vi "On Click Enumerate Cameras.vi"(8 "error in (no error)":errorcluster, 10 "Value":bool, 11 "App in":refnum<class "App.lvclass">) -> (0 "error out":errorcluster, 3 "App out":refnum<class "App.lvclass">)   [LabVIEW 2020, in "AR Example.lvlib" / "App.lvclass"]
uses:
  App.lvclass
  App.lvclass/App.ctl
  UI/UI.lvclass
  b0e96125-61a1-4303-b342-3e2cae2d3e9f.vi
  917a6586-ad63-4fd0-8dd0-0daf31f14cd0.vi
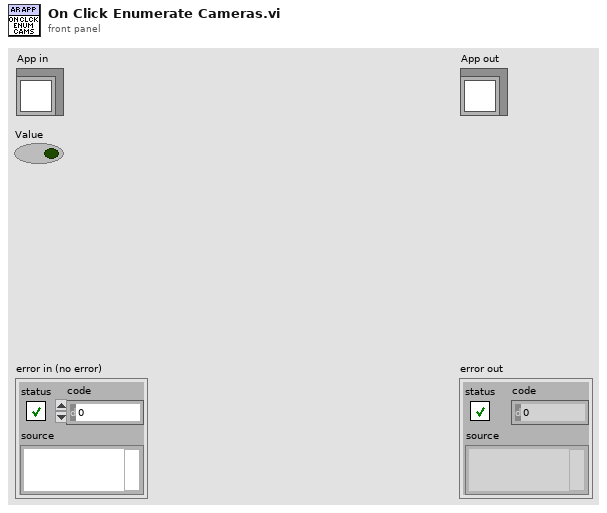
[diagram p1: front panel]
types:
  T1 = enum16{"Set UI Pre Enum", "Enumerate", "Update Lists", "Set UI Post Enum"}
  T2 = enum16{"Set UI Pre Enum", "Enumerate", "Update Lists", "Set UI Post Enum"}[]
  T3 = typedef "g_ar_toolkit.capture.lvlib/Stream.lvclass/Device Enumeration.ctl" = cluster{"Name":string, "Streams":set{T4}}
  T4 = typedef "g_ar_toolkit.capture.lvlib/Stream.lvclass/Stream Parameters.ctl" = cluster{"Width":u16, "Height":u16, "FPS":u8}
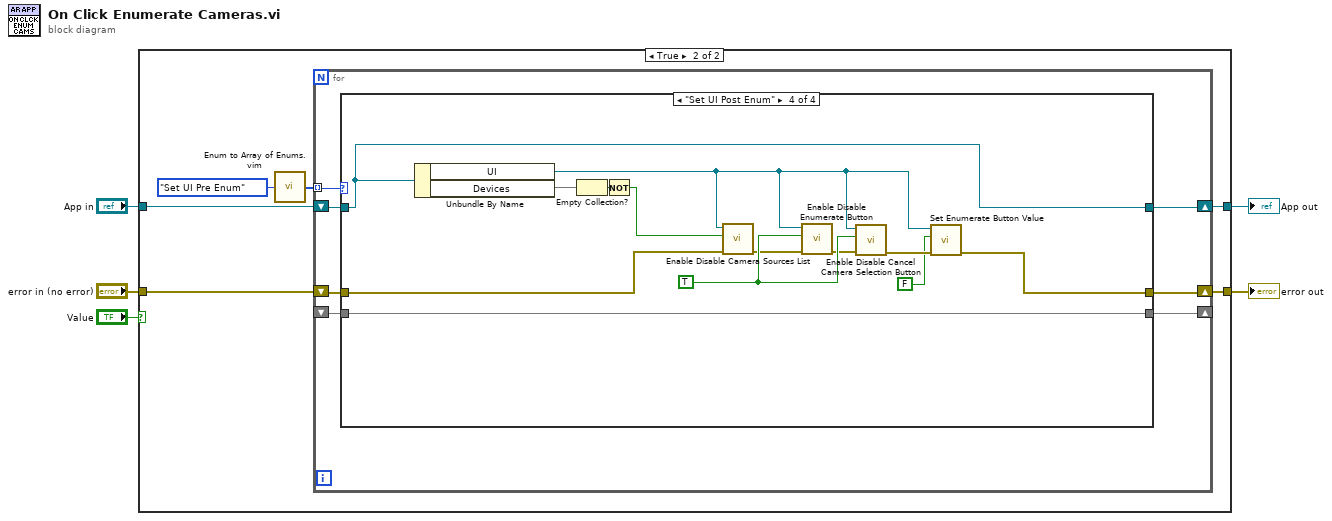
[diagram p0: block diagram]
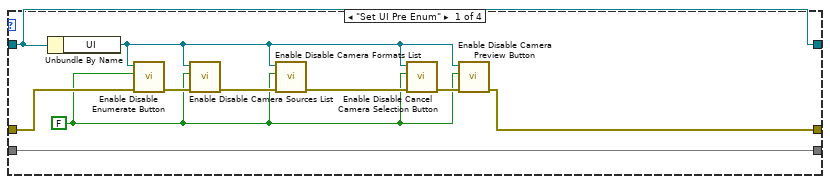
[diagram p3: hidden frame]
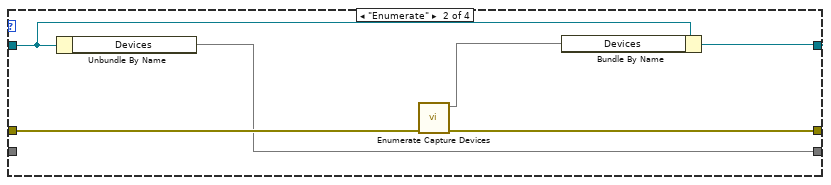
[diagram p4: hidden frame]
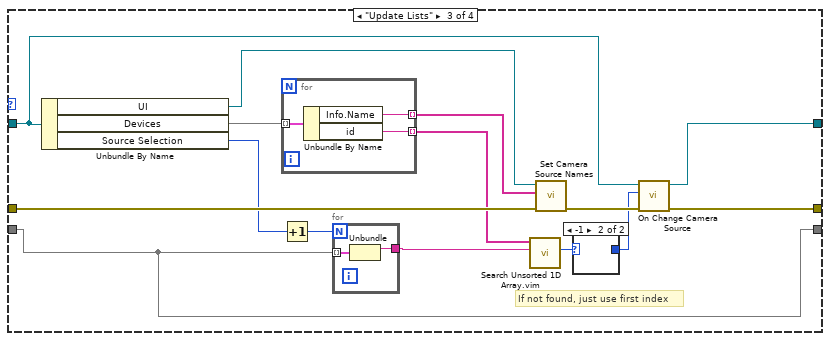
[diagram p5: hidden frame]
diagram:
  n1 = case shown="True" "Value" {
    tunnel: "App in" -> [w6 w13]
    tunnel: "error in (no error)" -> [w7 w12]
    tunnel: [w7 w11] -> w3
    tunnel: [w6 w10] -> w2
    frame False {
    }
    frame True {
      n2 = call "Enum to Array of Enums.vim"("enum"=T1."Set UI Pre Enum") -> ("array of enums"=w8:T2)
      n3 = for {
        shift-right: [w19] -> w11
        shift-left: w12 -> [w20]
        shift-right: [w16] -> w10
        shift-left: w13 -> [w18]
        tunnel: w8 -> [w17] mode=indexing
        shift-right: [w15] -> _
        shift-left: _ -> [w14]
        n4 = case shown="\"Set UI Post Enum\"" w17 {
          tunnel: w20 -> [w30 w36 w49 w60]
          tunnel: [w21 w33 w43 w64] -> w19
          tunnel: w18 -> [w26 w35 w45 w69]
          tunnel: [w26 w34 w44 w69] -> w16
          tunnel: [w25 w32 w51 w68] -> w15
          tunnel: w14 -> [w25 _ w51 w68]
          frame "Set UI Pre Enum" {
            w22 = FALSE ("Enable?")
            n5 = Unbundle By Name(w26) -> ("UI"=w23:refnum<class "UI.lvclass">)
            n6 = call-dynamic "Enable Disable Enumerate Button.vi"("error in (no error)"=w30, "Enable?"=w22, "UI in"=w23) -> ("error out"=w29:errorcluster)  [unwired: 8 in]
            n7 = call-dynamic "Enable Disable Camera Sources List.vi"("error in (no error)"=w29, "Enable?"=w22, "UI in"=w23) -> ("error out"=w28:errorcluster)  [unwired: 8 in]
            n8 = call-dynamic "Enable Disable Camera Formats List.vi"("error in (no error)"=w28, "Enable?"=w22, "UI in"=w23) -> ("error out"=w27:errorcluster)  [unwired: 8 in]
            n9 = call-dynamic "Enable Disable Cancel Camera Selection Button.vi"("error in (no error)"=w27, "Enable?"=w22, "UI in"=w23) -> ("error out"=w24:errorcluster)  [unwired: 8 in]
            n10 = call-dynamic "Enable Disable Camera Preview Button.vi"("error in (no error)"=w24, "Enable?"=w22, "UI in"=w23) -> ("error out"=w21:errorcluster)  [unwired: 8 in]
          }
          frame "Enumerate" {
            n11 = Unbundle By Name(w35) -> ("Devices"=w32:map{string, T3})
            n12 = call "Enumerate Capture Devices.vi"("error in (no error)"=w36) -> ("error out"=w33:errorcluster, "Devices"=w31:map{string, T3})  [unwired: 9 in]
            n13 = Bundle By Name(cluster=w35, "Devices"=w31) -> (w34:refnum<class "App.lvclass">)
          }
          frame "Update Lists" {
            # "If not found, just use first index"
            n14 = Unbundle By Name(w45) -> ("UI"=w48:refnum<class "UI.lvclass">, "Devices"=w50:map{string, T3}, "Source Selection"=w42:i32)
            n15 = for {
              tunnel: w50 -> [w57] mode=indexing
              tunnel: [w56] -> w47 mode=indexing
              tunnel: [w55] -> w41 mode=indexing
              n16 = Unbundle By Name(w57) -> ("Info.Name"=w56:string, "id"=w55:string)
            }
            n17 = Increment(x=w42) -> (x+1=w37:i32)
            n18 = for {
              N: w37 -> [_]
              tunnel: w51 -> [w54] mode=indexing
              tunnel: [w53] -> w40
              n19 = Unbundle(w54) -> ("id"=w53:string)  [unwired: 1 out]
            }
            n20 = call "Search Unsorted 1D Array.vim"("element"=w40, "unsorted 1D array"=w41) -> ("index of element"=w39:i32)  [unwired: 9 in]
            n21 = call-dynamic "Set Camera Source Names.vi"("error in (no error)"=w49, "Names"=w47, "UI in"=w48) -> ("error out"=w46:errorcluster)  [unwired: 8 in]
            n22 = case shown="-1" w39 {
              selector: w39 -> [w52 _]
              tunnel: [w52 _] -> w38
              frame Default {
              }
              frame -1 {
              }
            }
            n23 = call "On Change Camera Source.vi"("error in (no error)"=w46, "Selection"=w38, "App in"=w45) -> ("error out"=w43:errorcluster, "App out"=w44:refnum<class "App.lvclass">)  [unwired: 7 in]
          }
          frame "Set UI Post Enum" {
            w61 = TRUE ("Enable?")
            n24 = Unbundle By Name(w69) -> ("UI"=w63:refnum<class "UI.lvclass">, "Devices"=w67:map{string, T3})
            n25 = Empty Collection?(1:w67) -> (0:w66:bool)
            n26 = Not(x=w66) -> (.not. x?=w65:bool)
            n27 = call-dynamic "Enable Disable Camera Sources List.vi"("error in (no error)"=w60, "Enable?"=w65, "UI in"=w63) -> ("error out"=w59:errorcluster)  [unwired: 8 in]
            n28 = call-dynamic "Enable Disable Enumerate Button.vi"("error in (no error)"=w59, "Enable?"=w61, "UI in"=w63) -> ("error out"=w58:errorcluster)  [unwired: 8 in]
            n29 = call-dynamic "Enable Disable Cancel Camera Selection Button.vi"("error in (no error)"=w58, "Enable?"=w61, "UI in"=w63) -> ("error out"=w70:errorcluster)  [unwired: 8 in]
            n30 = call-dynamic "Set Enumerate Button Value.vi"("error in (no error)"=w70, "Values"=FALSE, "UI in"=w63) -> ("error out"=w64:errorcluster)  [unwired: 8 in]
          }
        }
      }
    }
  }
  "error out" <- w3
  "App out" <- w2
